vi "Group ID to Tree Items.vi"(8 "error in (no error)":errorcluster, 9 "Group ID":string, 11 "Application Data in":T2) -> (0 "error out":errorcluster, 1 "Settings":T1, 2 "Item":T1, 3 "Application Data out":T2)   [LabVIEW 2017, in "DSF Configuration Utility.lvlib"]
uses:
  DSF Configuration Utility.lvlib
  Main VI/Application Data.ctl
  VeriStand/Data Sharing Custom Device/Source/DSF Core.lvlibp/Classes/Configuration/Configuration Session.lvclass
  Main VI/View Mode.ctl
  Tree Item.ctl
  Tree Item Type.ctl
  VeriStand/Data Sharing Custom Device/Source/DSF Core.lvlibp/Classes/Configuration/Read Settings.vi
  VeriStand/Data Sharing Custom Device/Source/DSF Core.lvlibp/Classes/Configuration/Read Group.vi
panel:
  # "App\nData"
  # "App\nData"
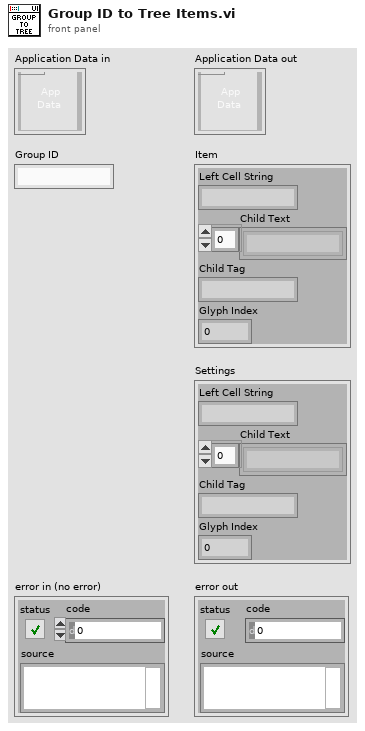
[diagram p1: front panel]
types:
  T1 = typedef "DSF Configuration Utility.lvlib/Tree Item.ctl" = cluster{"Left Cell String":string, "Child Text":string[], "Child Tag":string, "Glyph Index":i32}
  T2 = typedef "DSF Configuration Utility.lvlib/Application Data.ctl" = cluster{"Item Tree Control":refnum<vi>, "Value Tree Control":refnum<vi>, "DSF Refnum":refnum<class "Configuration Session.lvclass">, "Top-Level VI":refnum<vi>, "View State":T3, "menu reference":refnum<k9>}
  T3 = typedef "DSF Configuration Utility.lvlib/View Mode.ctl" = enum16{"Tree", "List"}
  T4 = typedef "DSF Configuration Utility.lvlib/Tree Item Type.ctl" = enum16{"Plugin", "Group", "Transfer", "Channel", "Setting"}
  T5 = typedef "DSF Core.lvlibp/DSF Group Info.ctl" = cluster{"direction":T6, "timing":T7, "transfer ids":string[], "settings id":string, "thread":i32, "timeout behavior":T8}
  T6 = typedef "DSF Core.lvlibp/DSF Direction.ctl" = enum8{"Tx", "Rx"}
  T7 = typedef "DSF Core.lvlibp/DSF Timing Info.ctl" = cluster{"priority":u64, "decimation":u64, "offset":u64}
  T8 = typedef "DSF Core.lvlibp/DSF Timeout Behavior.ctl" = enum8{"Increment Late Count", "Throw Error"}
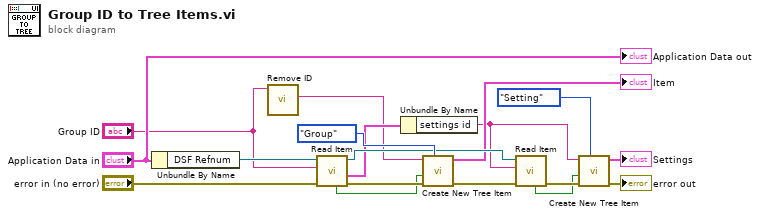
[diagram p0: block diagram]
diagram:
  n1 = Unbundle By Name("Application Data in") -> ("DSF Refnum"=w8:refnum<class "Configuration Session.lvclass">)
  n2 = call "Remove ID.vi"("id string"="Group ID") -> ("name"=w1:string)  [unwired: 8 in, 2 out]
  n3 = call-poly "Read Item.vi"("error in (no error)"="error in (no error)", "Group ID"="Group ID", "Configuration Session in"=w8) -> ("error out"=w14:errorcluster, "value"=w11:T5, "Configuration Session out"=w13:refnum<class "Configuration Session.lvclass">, "found?"=w4:bool)  [unwired: 5 in]
  n4 = Unbundle By Name(w11) -> ("settings id"=w5:string)
  n5 = call "Create New Tree Item.vi"("Item Type"=Tree_Item_Type."Group", "error in"=w14, "found?"=w4, "Left Cell String"=w1) -> ("error out"=w15:errorcluster, "Item"=→"Item":T1)  [unwired: 6 in]
  n6 = call-poly "Read Item.vi"("error in (no error)"=w15, "Settings ID"=w5, "Configuration Session in"=w13) -> ("error out"=w16:errorcluster, "found?"=w3:bool)  [unwired: 5 in, 2 out]
  n7 = call "Create New Tree Item.vi"("Item Type"=Tree_Item_Type."Setting", "error in"=w16, "found?"=w3, "Left Cell String"=w5) -> ("error out"=→"error out":errorcluster, "Item"=→"Settings":T1)  [unwired: 6 in]
  "Application Data out" <- "Application Data in"
